vi "Calibrate.vi"(8 "error in (no error)":errorcluster, 11 "Insight in":refnum<class "Insight.lvclass">) -> (0 "error out":errorcluster, 3 "Insight out":refnum<class "Insight.lvclass">)   [LabVIEW 2015, in "Insight.lvclass"]
uses:
  Insight.lvclass
  Insight.lvclass/Insight.ctl
  Laser.lvclass
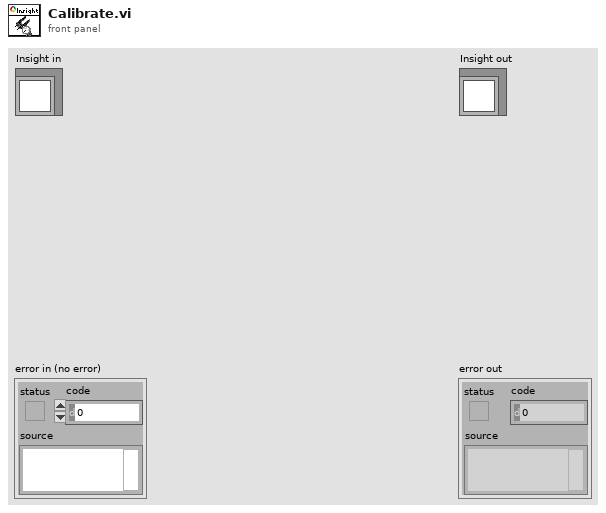
[diagram p1: front panel]
types:
  T1 = typedef "Telnet Session.ctl" = refnum<k1>
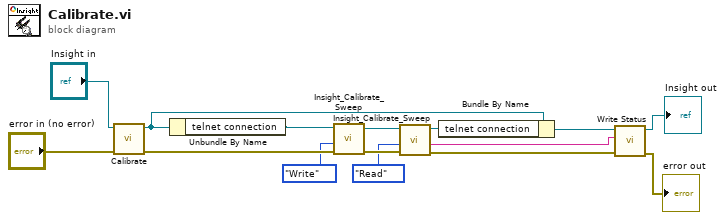
[diagram p0: block diagram]
diagram:
  n1 = call-parent "Calibrate.vi"("error in (no error)"="error in (no error)", "Laser in"="Insight in") -> ("error out"=w13:errorcluster, "Laser out"=w5:refnum<class "Insight.lvclass">)  [unwired: 8 in]
  n2 = Unbundle By Name(w5) -> ("telnet connection"=w11:T1)
  n3 = call "Insight_Calibrate_Sweep.vi"("error in (no error)"=w13, "Mode (Read / Write)"=enum8{"Write", "Read"}."Write", "telnet connection"=w11) -> ("error out"=w10:errorcluster, "telnet  connection out"=w9:T1)  [unwired: 6 in, 1 out]
  n4 = call "Insight_Calibrate_Sweep.vi"("error in (no error)"=w10, "Mode (Read / Write)"=enum8{"Write", "Read"}."Read", "telnet connection"=w9) -> ("error out"=w3:errorcluster, "response data"=w6:string, "telnet  connection out"=w7:T1)  [unwired: 6 in]
  n5 = Bundle By Name(cluster=w5, "telnet connection"=w7) -> (w4:refnum<class "Insight.lvclass">)
  n6 = call-dynamic "Write Status.vi"("error in (no error)"=w3, "Status"=w6, "Laser in"=w4) -> ("error out"=→"error out":errorcluster, "Laser out"=→"Insight out":refnum<class "Insight.lvclass">)  [unwired: 7 in]
